vi "Color Test.vi"() -> ()   [LabVIEW 2015]
panel:
  in  "OK":bool
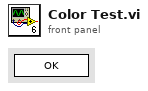
[diagram p1: front panel]
types:
  T1 = enum32{"invalid app kind", "Development System", "Run Time System", "Student Edition", "Embedded LabVIEW", "Evaluation", "Custom"}
  T2 = enum32{"Invalid", "Standard", "Closed", "Hidden", "Minimized", "Maximized"}
  T3 = cluster{"Core":cluster{"Current VI Reference":refnum<vi>, "Close Panel on Exit?":bool}, "Color data":cluster{"Attribute":string, "Color":u32}[][]}
  T4 = cluster{"Current VI Reference":refnum<vi>, "Close Panel on Exit?":bool}
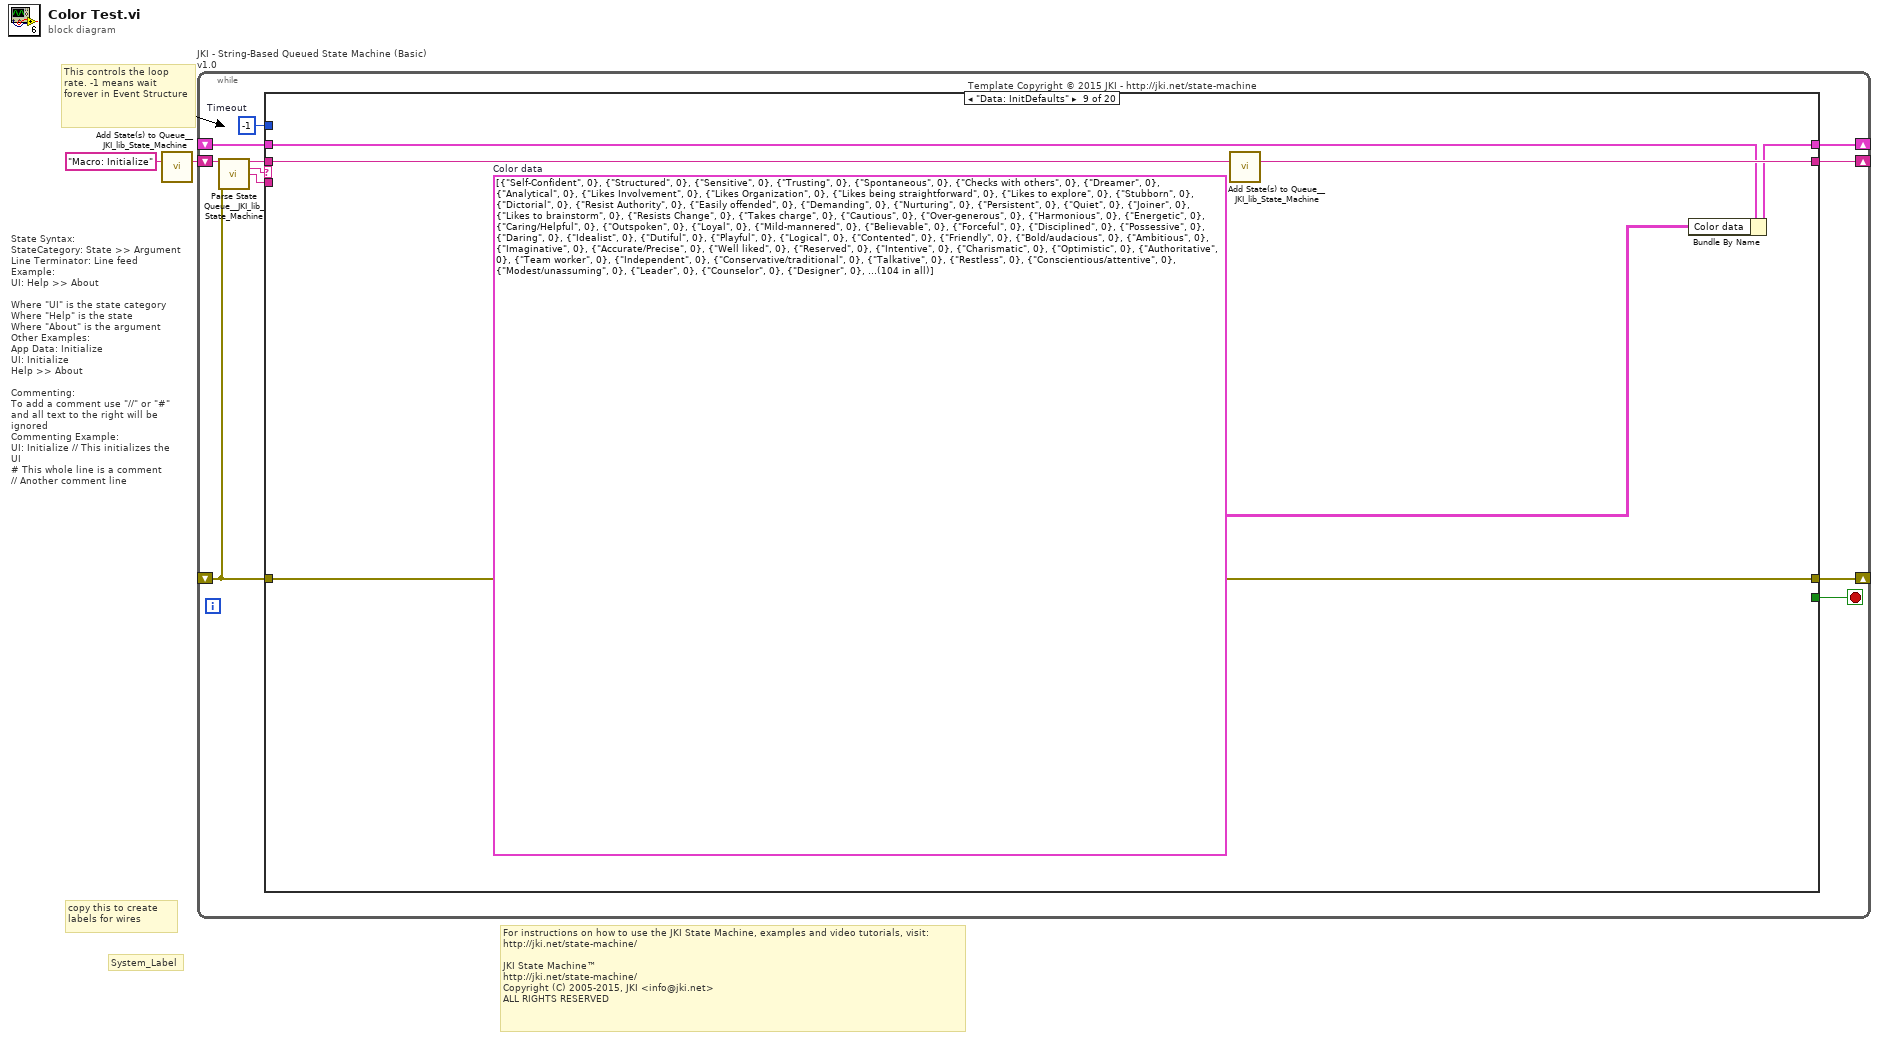
[diagram p0: block diagram]
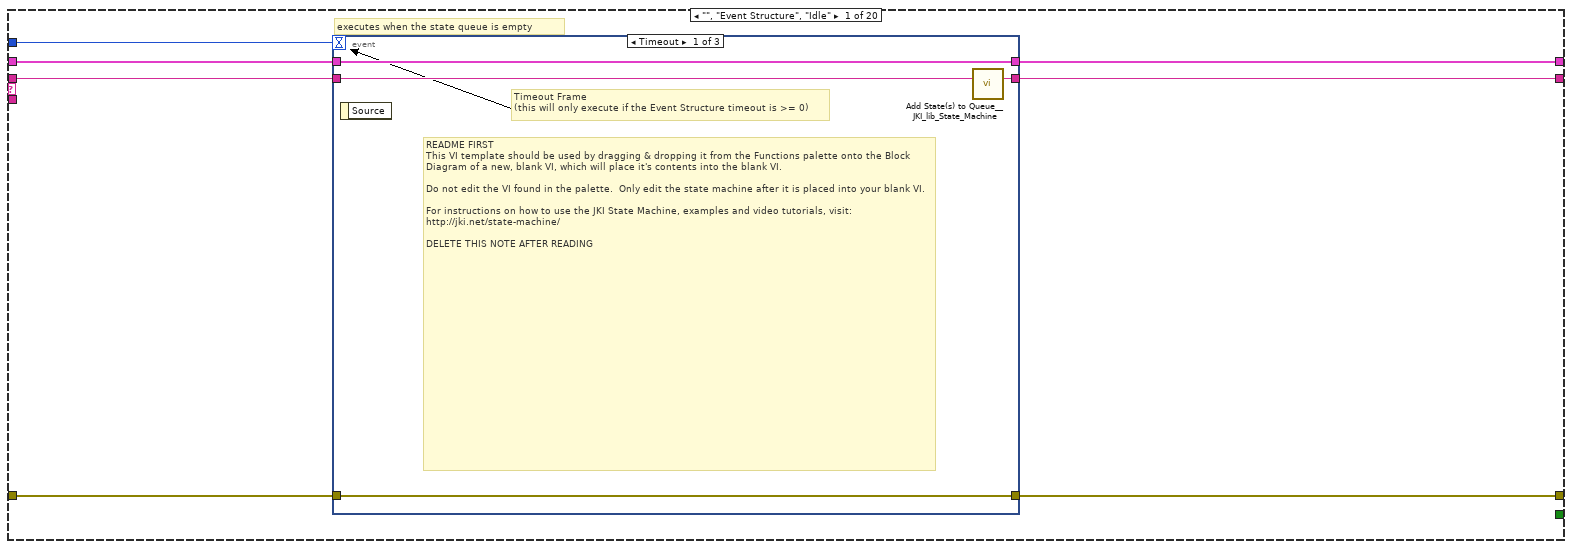
[diagram p2: hidden frame]
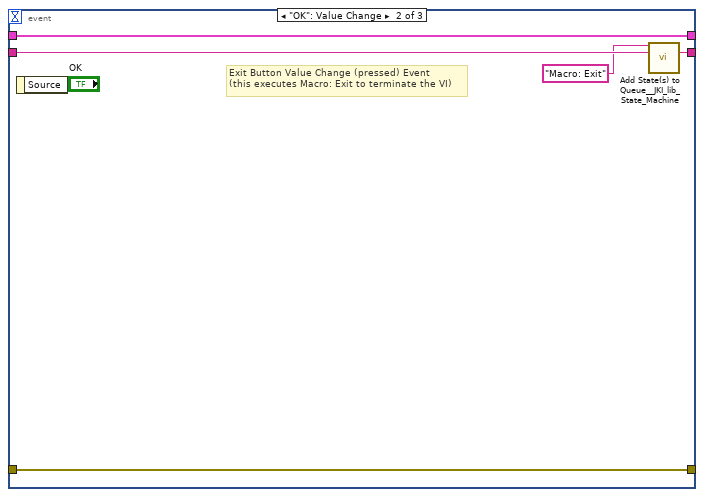
[diagram p3: hidden frame]
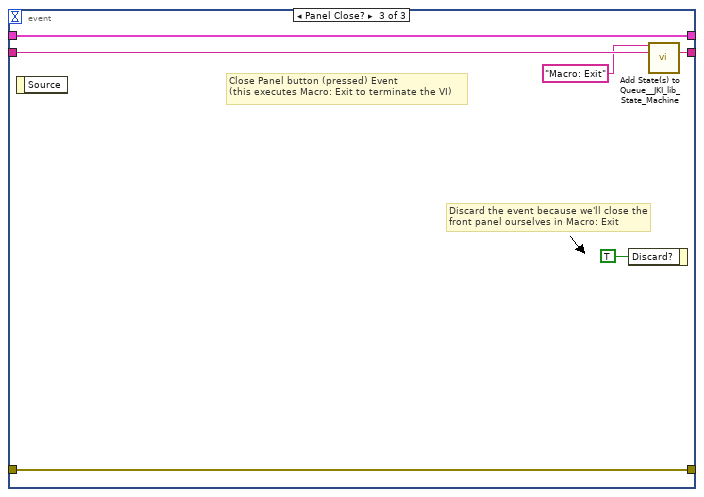
[diagram p4: hidden frame]
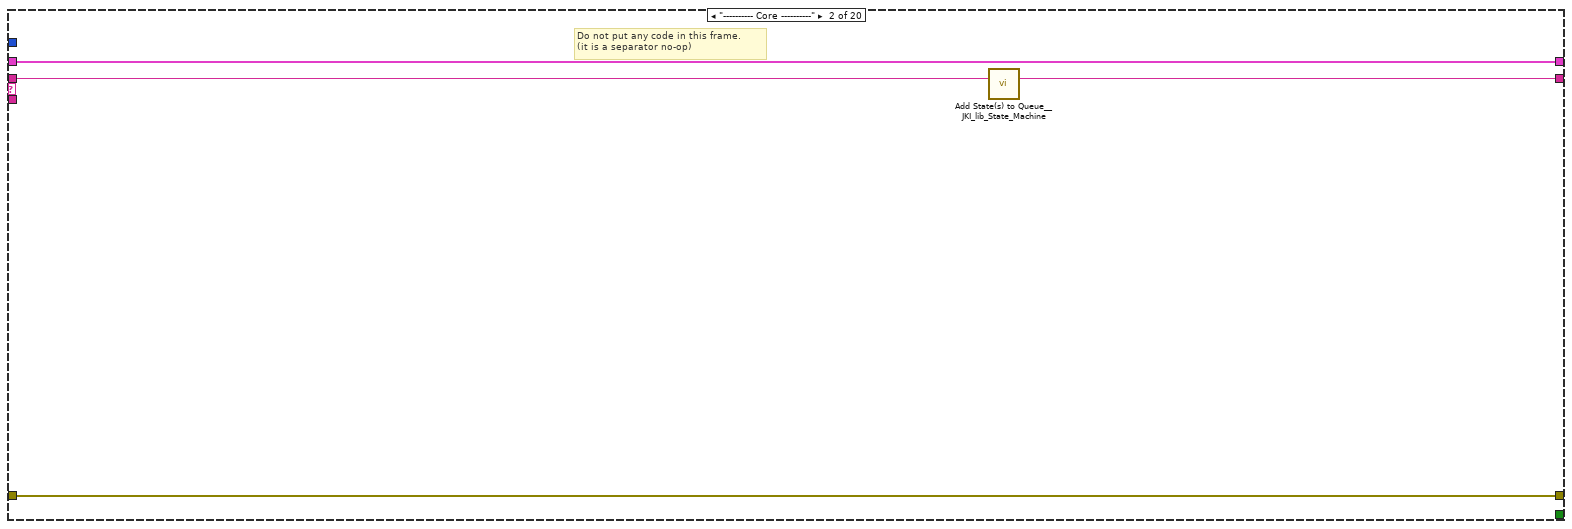
[diagram p5: hidden frame]
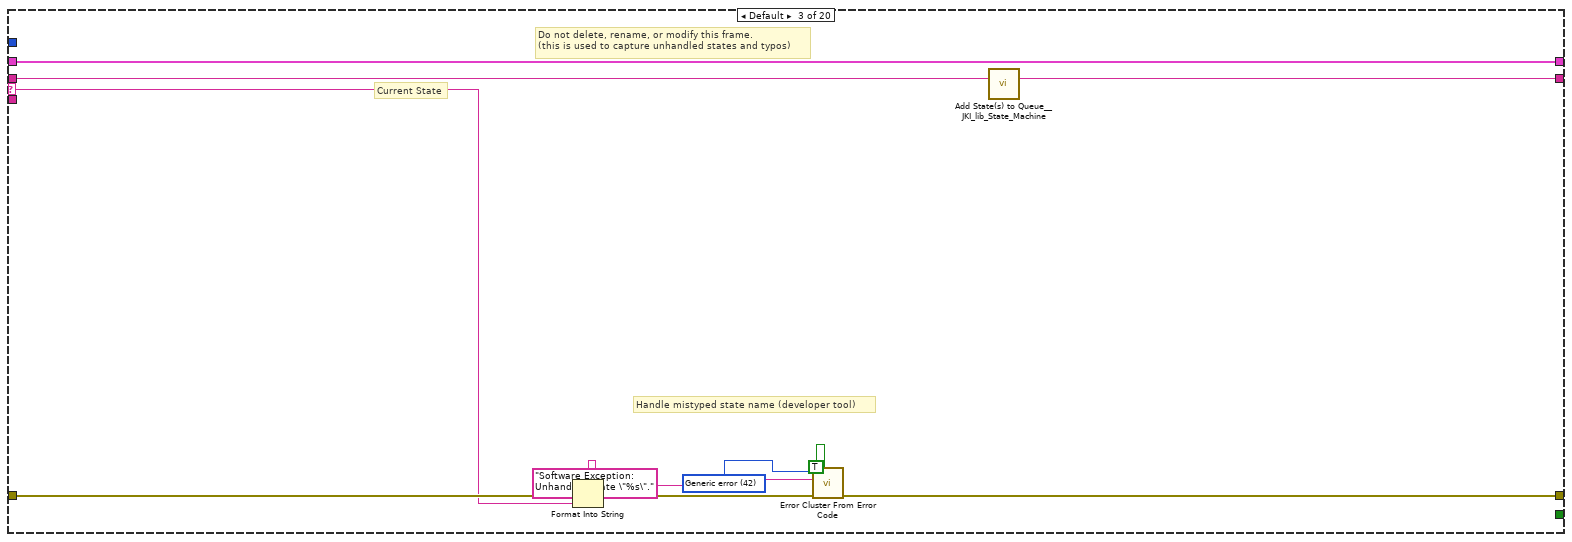
[diagram p6: hidden frame]
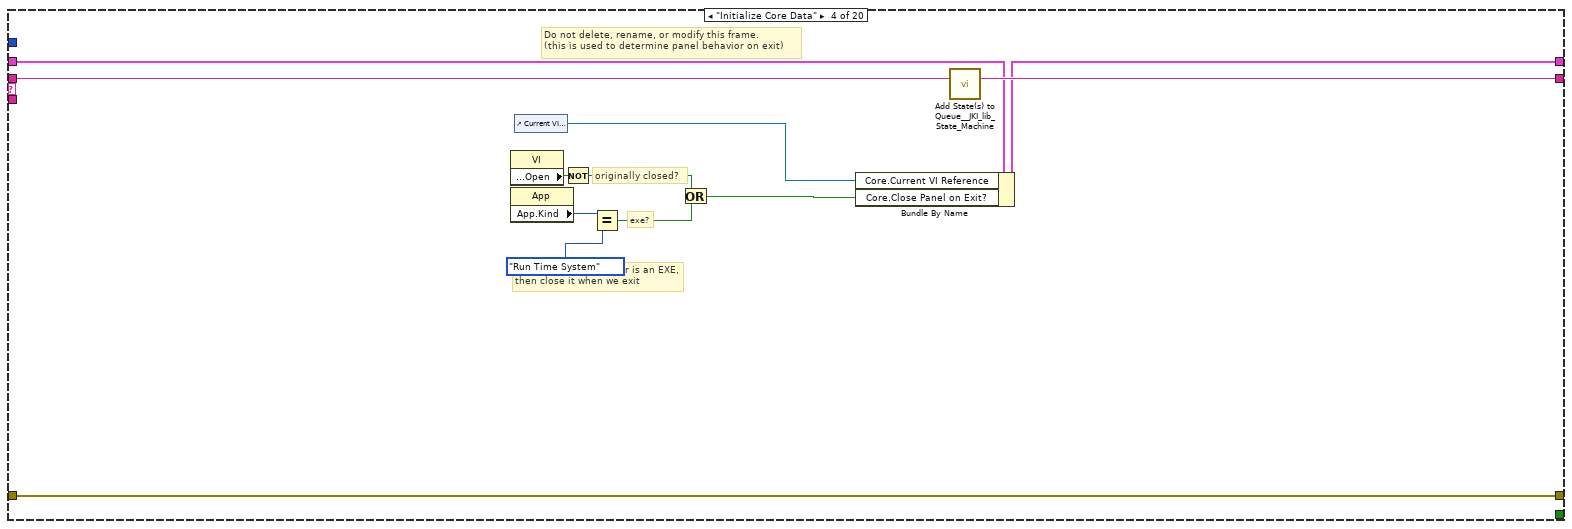
[diagram p7: hidden frame]
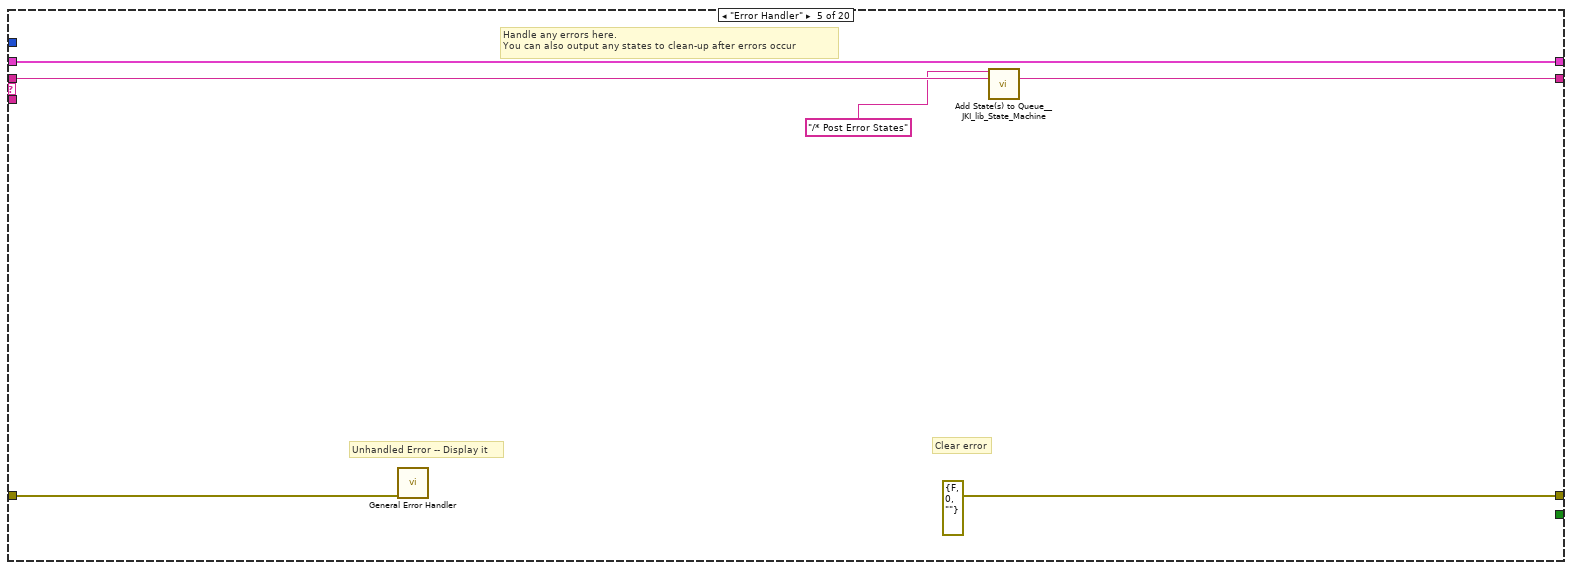
[diagram p8: hidden frame]
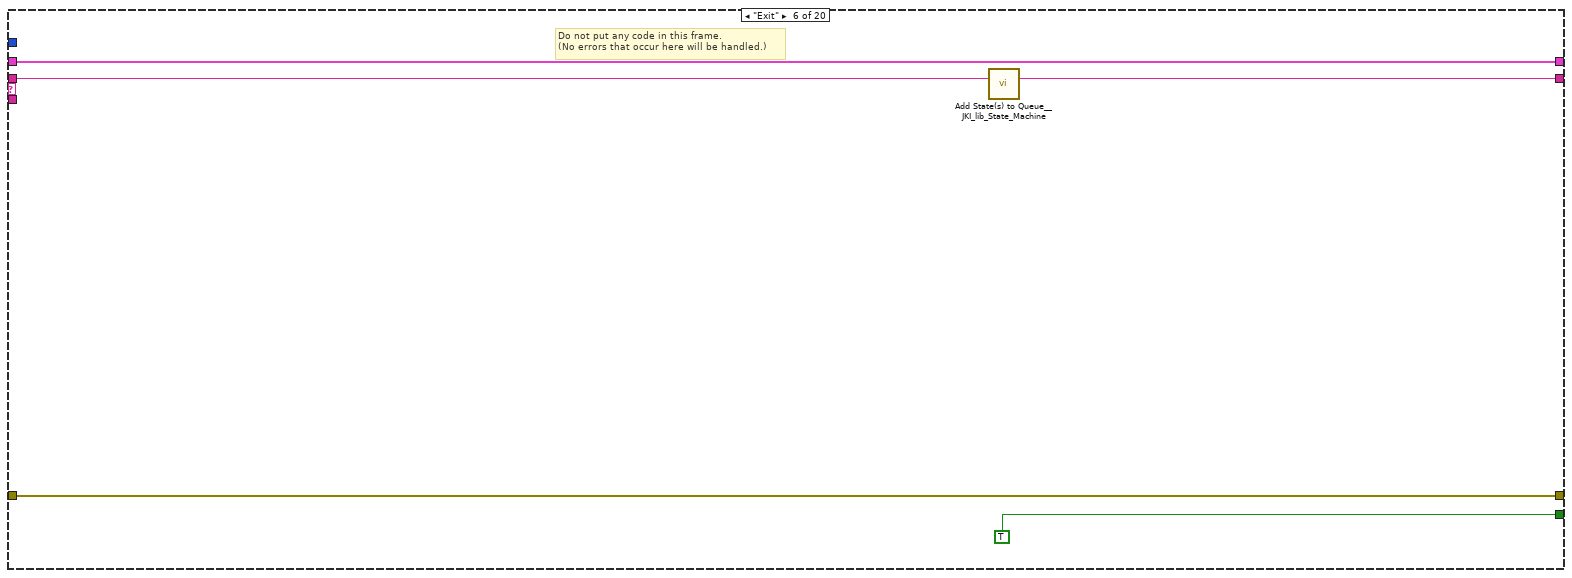
[diagram p9: hidden frame]
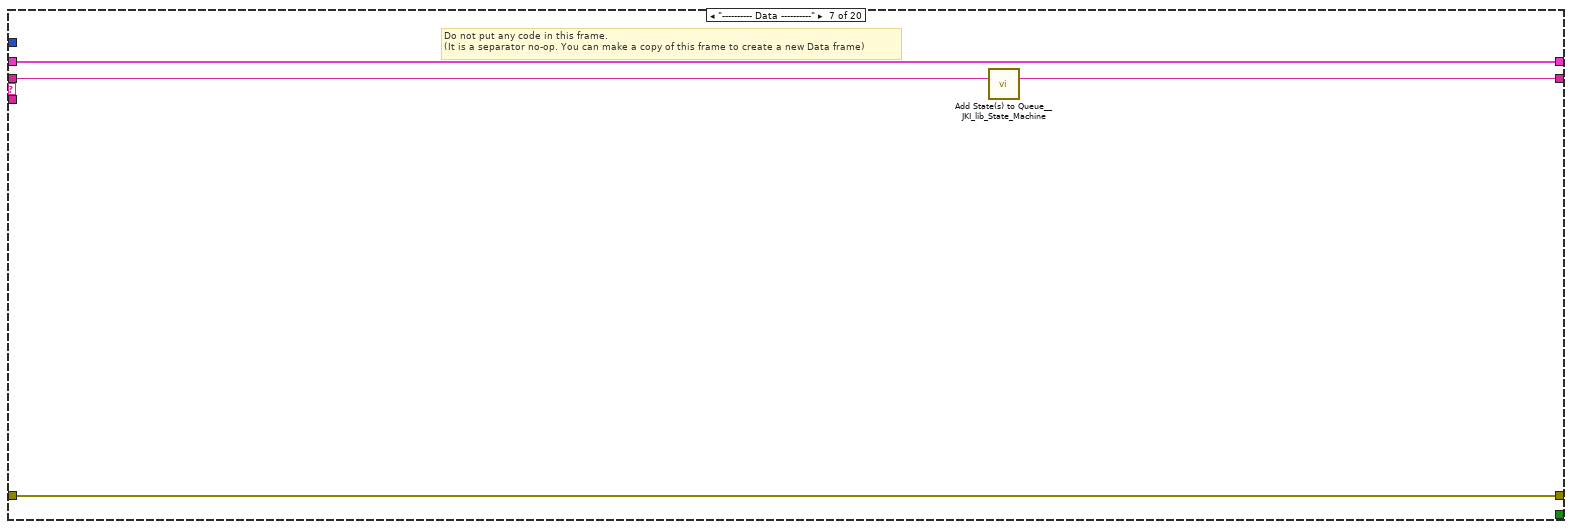
[diagram p10: hidden frame]
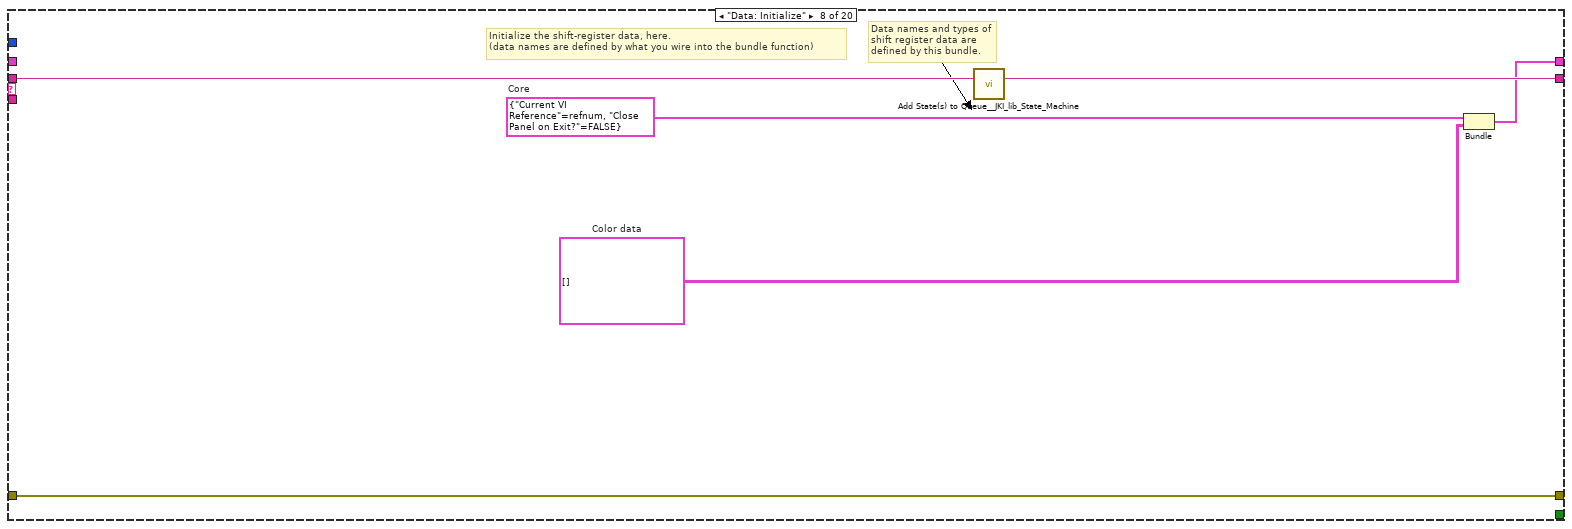
[diagram p11: hidden frame]
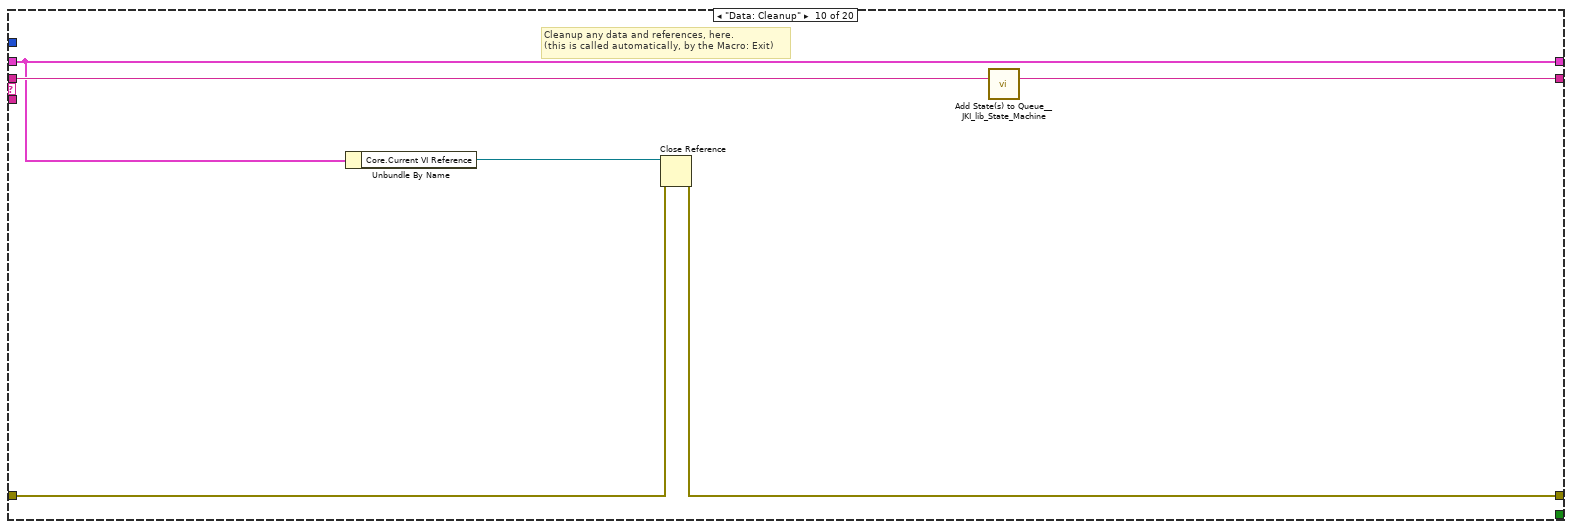
[diagram p12: hidden frame]
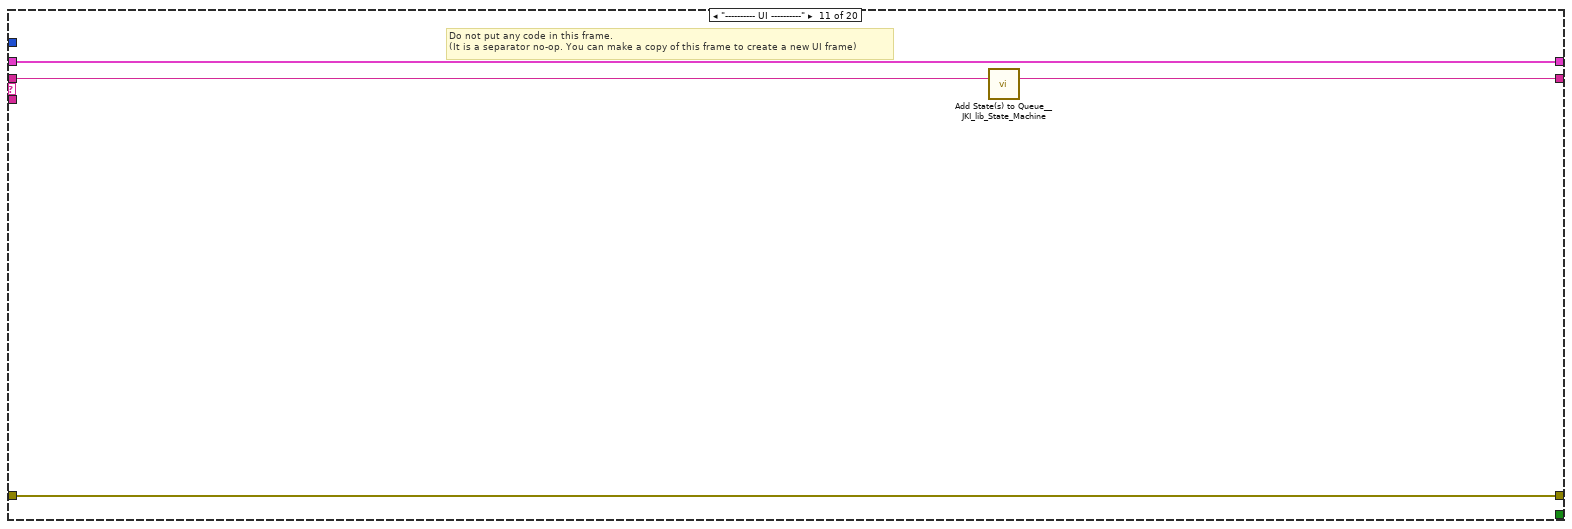
[diagram p13: hidden frame]
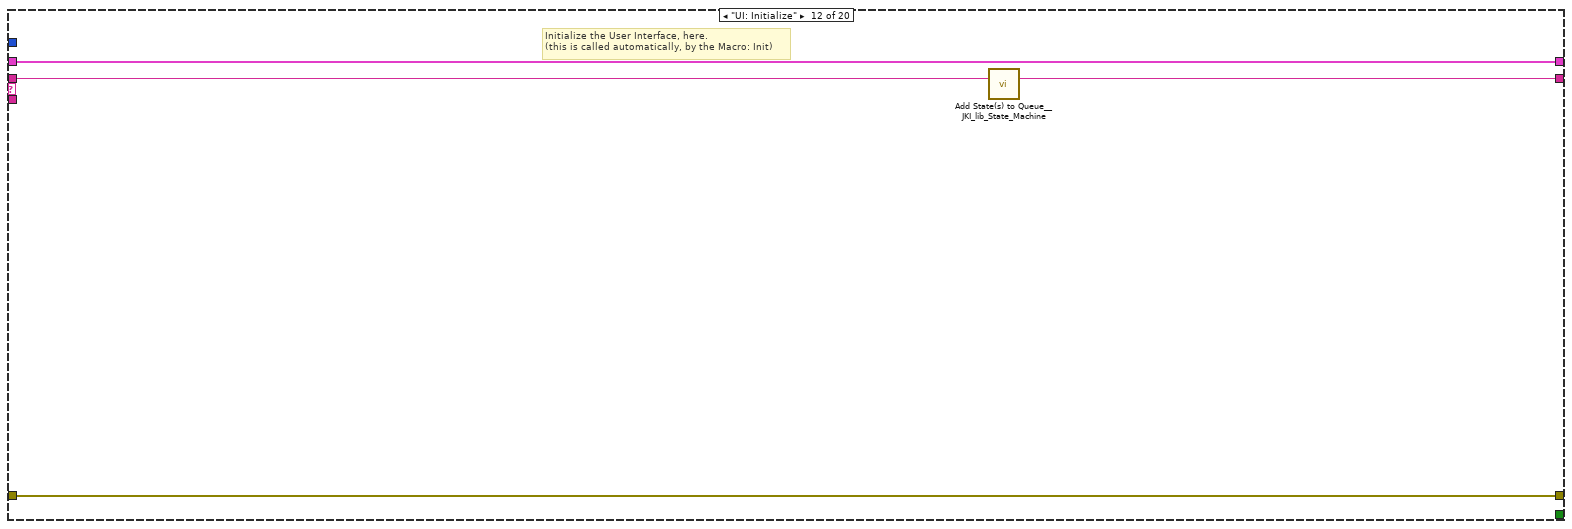
[diagram p14: hidden frame]
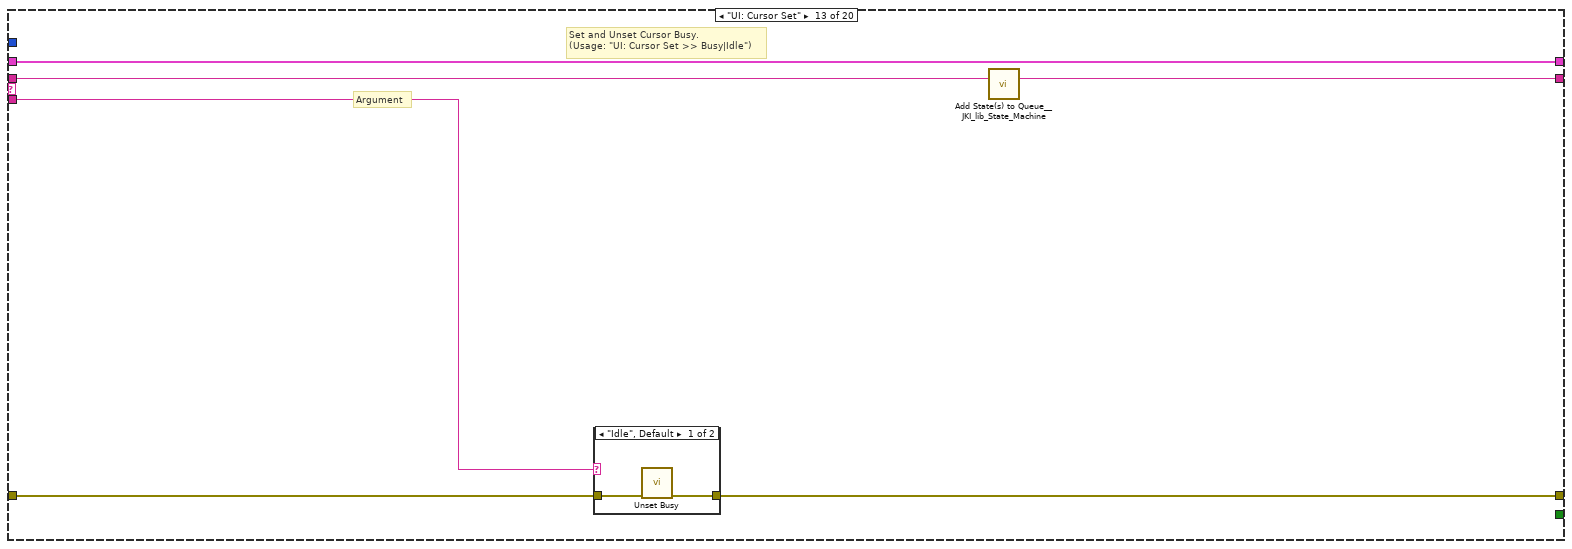
[diagram p15: hidden frame]
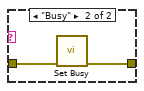
[diagram p16: hidden frame]
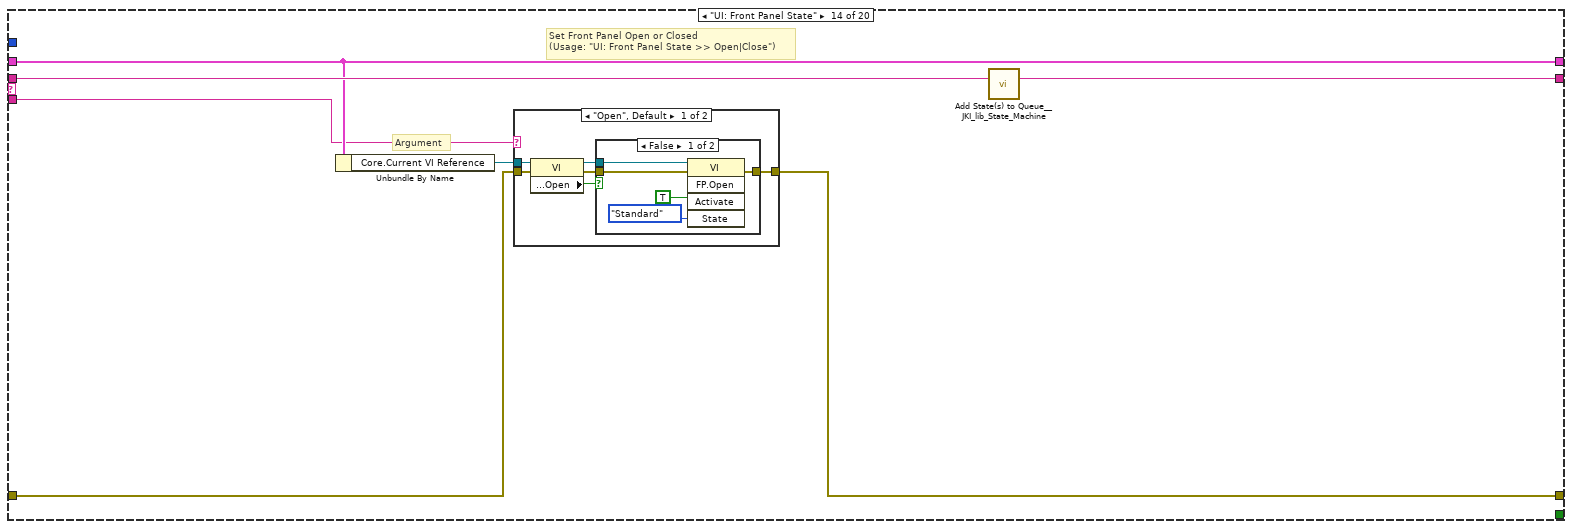
[diagram p17: hidden frame]
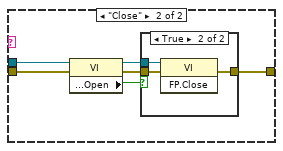
[diagram p19: hidden frame]
diagram:
  # "For instructions on how to use the JKI State Machine, examples and video tutorials, visit:\nhttp://jki.net/state-machine/\n\nJKI State Machine™\nhttp://jki.net/state-machine/\nCopyright (C) 2005-2015, JKI <info@jki.net>\nALL RIGHTS RESERVED"
  # "State Syntax:\nStateCategory: State >> Argument\nLine Terminator: Line feed\nExample:\nUI: Help >> About\n\nWhere \"UI\" is the state category\nWhere \"Help\" is the state\nWhere \"About\" is the argument\nOther Examples:\nApp Data: Initialize\nUI: Initialize\nHelp >> About\n\nCommenting:\nTo add a comment use \"//\" or \"#\" and all text to the right will be ignored\nCommenting Example:\nUI: Initialize // This initializes the UI\n# This whole line is a comment\n// Another comment line"
  # "copy this to create labels for wires"
  # "This controls the loop rate. -1 means wait forever in Event Structure"
  # "System_Label"
  n1 = call <vilib>:"Add State(s) to Queue__JKI_lib_State_Machine.vi"("State(s) in (\"\")"="Macro: Initialize") -> ("States Out"=w2:string)  [unwired: 14 in]
  n2 = while "JKI - String-Based Queued State Machine (Basic) v1.0" {
    shift-right: [w6] -> _
    shift-left: _ -> [w5]
    shift-right: [w9] -> _
    shift-left: _ -> [w3]
    shift-right: [w8] -> _
    shift-left: w2 -> [w10]
    stop <- w7 stop-if-true
    w4 = -1  # Timeout
    # "Template Copyright © 2015 JKI - http://jki.net/state-machine"
    n3 = call <vilib>:"Parse State Queue__JKI_lib_State_Machine.vi"("State Queue"=w10, "Error In (no error)"=w3) -> ("Remaining States"=w12:string, "Current State"=w13:string, "Arguments"=w11:string)  [unwired: 11 in]
    n4 = case shown="\"Data: InitDefaults\"" w13 {
      selector: w13 -> [_ _ w40 _ _ _ _ _ _ _ _ _ _ _ _ _ _ _ _ _]
      tunnel: w12 -> [w20 w39 w44 w62 w68 w73 w77 w83 w89 w95 w99 w103 w109 w120 w146 w151 w161 w165 w169 w173]
      tunnel: w11 -> [_ _ _ _ _ _ _ _ _ _ _ _ w104 w114 _ _ _ _ _ _]
      tunnel: w5 -> [w18 w36 w42 w53 w65 w71 w74 _ w86 w90 w96 w101 w107 w116 w143 w148 w158 w162 w166 w170]
      tunnel: [w17 w37 w46 w59 errorcluster {"status"=FALSE, "code"=0, "source"=""} ("error out") w70 w75 w80 w87 w91 w97 w100 w105 w117 w144 w149 w159 w163 w167 w171] -> w9
      tunnel: w3 -> [w16 w37 w45 w59 w64 w70 w75 w80 w87 w92 w97 w100 w106 w118 w144 w149 w159 w163 w167 w171]
      tunnel: [w19 w38 w43 w61 w67 w72 w76 w82 w88 w94 w98 w102 w108 w119 w145 w150 w160 w164 w168 w172] -> w8
      tunnel: [_ _ _ _ _ TRUE _ _ _ _ _ _ _ _ _ _ _ _ _ _] -> w7
      tunnel: [w15 w36 w42 w60 w65 w71 w74 w81 w85 w90 w96 w101 w107 w116 w143 w148 w158 w162 w166 w170] -> w6
      tunnel: w4 -> [w14 _ _ _ _ _ _ _ _ _ _ _ _ _ _ _ _ _ _ _]
      frame "", "Event Structure", "Idle" {
        # "executes when the state queue is empty"
        n5 = event shown="[0] Timeout" {
          selector: _ -> [_ _ _]
          dyn-events: _ -> [_ _ _]
          timeout: w14 -> [_ _ _]
          tunnel: w20 -> [w24 w29 w35]
          tunnel: [w23 w28 w34] -> w19
          tunnel: w18 -> [w21 w26 w32]
          tunnel: [w22 w27 w33] -> w17
          tunnel: w16 -> [w22 w27 w33]
          tunnel: [w21 w26 w32] -> w15
          event Timeout {
            # "README FIRST\nThis VI template should be used by dragging & dropping it from the Functions palette onto the Block Diagram of a new, blank VI, which will place it's contents into the blank VI.\n\nDo not edit the VI found in the palette.  Only edit the state machine after it is placed into your blank VI.\n\nFor instructions on how to use the JKI State Machine, examples and video tutorials, visit:\nhttp://jki.net/state-machine/\n\nDELETE THIS NOTE AFTER READING"
            # "Timeout Frame\n(this will only execute if the Event Structure timeout is >= 0)"
            n6 = event-data() -> ()  [unwired: 1 in, 1 out]
            n7 = call <vilib>:"Add State(s) to Queue__JKI_lib_State_Machine.vi"("State(s) in (\"\")"=w24) -> ("States Out"=w23:string)  [unwired: 14 in]
          }
          event "OK": Value Change {
            # "Exit Button Value Change (pressed) Event\n(this executes Macro: Exit to terminate the VI)"
            n8 = event-data() -> ()  [unwired: 1 in, 1 out]
            n9 = call <vilib>:"Add State(s) to Queue__JKI_lib_State_Machine.vi"("State(s) in Front (\"\")"="Macro: Exit", "State(s) in (\"\")"=w29) -> ("States Out"=w28:string)  [unwired: 13 in]
          }
          event Panel Close? {
            # "Discard the event because we'll close the front panel ourselves in Macro: Exit"
            # "Close Panel button (pressed) Event\n(this executes Macro: Exit to terminate the VI)"
            n10 = event-data() -> ()  [unwired: 1 in, 1 out]
            n11 = event-data("Discard?"=TRUE) -> ()  [unwired: 1 in, 1 out]
            n12 = call <vilib>:"Add State(s) to Queue__JKI_lib_State_Machine.vi"("State(s) in Front (\"\")"="Macro: Exit", "State(s) in (\"\")"=w35) -> ("States Out"=w34:string)  [unwired: 13 in]
          }
        }
      }
      frame "---------- Core ----------" {
        # "Do not put any code in this frame.\n(it is a separator no-op)"
        n13 = call <vilib>:"Add State(s) to Queue__JKI_lib_State_Machine.vi"("State(s) in (\"\")"=w39) -> ("States Out"=w38:string)  [unwired: 14 in]
      }
      frame Default {
        w49 = 42 items=["No error", "Argument error", "Memory is full", "Out of zone", "End of file", "File already open", "Generic file I/O error", "File not found", "File permission error", "Disk is full", "Duplicate path", "Too many files open", "System feature not enabled", "Resource file not found", "Cannot add resource", "Resource not found", "Image not found", "Image memory error", "Pen does not exist", "Config type invalid", "Config token not found", "Config parse error", "Config memory error", "Bad external code format", "Bad external code offset", "External code not present", "Null window", "Destroy window error", "Null menu", "Print aborted", "Bad print record", "Print driver error", "Windows error during printing", "Memory error during printing", "Print dialog error", "Generic print error", "Invalid device refnum", "Device not found", "Device parameter error", "Device unit error", "Cannot open device", "Device call aborted", "Generic error", "Cancelled by user", "Object ID too low", "Object ID too high", "Object not in heap", "Unknown heap", "Unknown object (invalid DefProc)", "Unknown object (DefProc not in table)", "Message out of range", "Invalid (null) method", "Unknown message", "Manager call not supported", "Bad address", "Network operation in progress", "Network operation timed out", "Connection is busy", "Network attribute not supported", "Network error", "Address in use", "System out of memory", "Connection aborted", "Connection refused", "Not connected", "Already connected", "Connection closed", "Initialization error (interapplication manager)", "Bad occurrence", "Wait on unbound occurrence handler", "Occurrence queue overflow", "Datalog type conflict", "Unused", "Unrecognized type (interapplication manager)", "Memory corrupt", "Failed to make temporary DLL", "Old CIN version", "Drag socket not found", "Failed to load drop-object", "Failed to register OLE object", "Failed to release OLE object", "Format specifier type mismatch", "Unknown format specifier", "Too few format specifiers", "Too many format specifiers", "Scan failed", "Newer CIN version", "Error converting to variant", "Runtime menu error", "Password tampered", "Variant attribute not found", "Incompatible variant data type", "Event data is not available", "Event Store is not present", "Occurrence is not found", "Event Queue is not created", "Event info is not available", "Refnum passed is NULL", "Error retrieving Class GUID", "Error retrieving CoClass GUID", "Error retrieving TypeLib GUID.", "Bad built application magic bytes.", "Specific driver is different from the specific driver associated with the Logical Name.", "There is no session opened to the class driver.", "Max Error", "MAX - Error with config objects", "MAX - Error loading configuration", "MAX - Group not supported"]
        # "Current State"
        # "Do not delete, rename, or modify this frame.\n(this is used to capture unhandled states and typos)"
        # "Handle mistyped state name (developer tool)"
        n14 = Format Into String(format string="Software Exception: Unhandled State \"%s\"." ("message"), error in=w45, w40) -> (resulting string=w48:string, error out=w47:errorcluster)  [unwired: 1 in]
        n15 = call <vilib>:"Error Cluster From Error Code.vi"("show call chain? (False)"=TRUE, "error in (no error)"=w47, "error message (\"\")"=w48, "error code (0)"=w49) -> ("error out"=w46:errorcluster)  [unwired: 5 in]
        n16 = call <vilib>:"Add State(s) to Queue__JKI_lib_State_Machine.vi"("State(s) in (\"\")"=w44) -> ("States Out"=w43:string)  [unwired: 14 in]
      }
      frame "Initialize Core Data" {
        # "Do not delete, rename, or modify this frame.\n(this is used to determine panel behavior on exit)"
        # "originally closed?"
        # "exe?"
        # "If panel starts closed or is an EXE, then close it when we exit"
        n17 = property class="VI"() -> ("Front Panel.Open"=w58:bool)  [unwired: 2 in, 2 out]
        n18 = property class="App"() -> ("App.Kind"=w57:T1)  [unwired: 2 in, 2 out]
        n19 = control-ref of="Current VI Reference"() -> (w51:refnum<vi>)
        n20 = Not(x=w58) -> (.not. x?=w55:bool)
        n21 = Equal?(x=w57, y=T1."Run Time System" ("Application:Kind")) -> (x = y?=w54:bool)
        n22 = Or(x=w55, y=w54) -> (x .or. y?=w52:bool)
        n23 = Bundle By Name(cluster=w53, "Core.Current VI Reference"=w51, "Core.Close Panel on Exit?"=w52) -> (w60:T3)
        n24 = call <vilib>:"Add State(s) to Queue__JKI_lib_State_Machine.vi"("State(s) in (\"\")"=w62) -> ("States Out"=w61:string)  [unwired: 14 in]
      }
      frame "Error Handler" {
        # "Unhandled Error -- Display it"
        # "Handle any errors here.\nYou can also output any states to clean-up after errors occur"
        # "Clear error"
        n25 = call <vilib>:"General Error Handler.vi"("error in (no error)"=w64) -> ()  [unwired: 10 in, 5 out]
        n26 = call <vilib>:"Add State(s) to Queue__JKI_lib_State_Machine.vi"("State(s) in Front (\"\")"="/* Post Error States", "State(s) in (\"\")"=w68) -> ("States Out"=w67:string)  [unwired: 13 in]
      }
      frame "Exit" {
        # "Do not put any code in this frame.\n(No errors that occur here will be handled.)"
        n27 = call <vilib>:"Add State(s) to Queue__JKI_lib_State_Machine.vi"("State(s) in (\"\")"=w73) -> ("States Out"=w72:string)  [unwired: 14 in]
      }
      frame "---------- Data ----------" {
        # "Do not put any code in this frame.\n(It is a separator no-op. You can make a copy of this frame to create a new Data frame)"
        n28 = call <vilib>:"Add State(s) to Queue__JKI_lib_State_Machine.vi"("State(s) in (\"\")"=w77) -> ("States Out"=w76:string)  [unwired: 14 in]
      }
      frame "Data: Initialize" {
        w78 = cluster{"Attribute":string, "Color":u32}[][] []  # Color data
        w79 = T4 {"Current VI Reference"=refnum, "Close Panel on Exit?"=FALSE}  # Core
        # "Data names and types of shift register data are defined by this bundle."
        # "Initialize the shift-register data, here.\n(data names are defined by what you wire into the bundle function)"
        n29 = call <vilib>:"Add State(s) to Queue__JKI_lib_State_Machine.vi"("State(s) in (\"\")"=w83) -> ("States Out"=w82:string)  [unwired: 14 in]
        n30 = Bundle("Core"=w79, "Color data"=w78) -> (w81:T3)  [unwired: 1 in]
      }
      frame "Data: InitDefaults" {
        w84 = cluster{"Attribute":string, "Color":u32}[][] [[{"Attribute"="Self-Confident", "Color"=0}, {"Attribute"="Structured", "Color"=0}, {"Attribute"="Sensitive", "Color"=0}, {"Attribute"="Trusting", "Color"=0}], [{"Attribute"="Spontaneous", "Color"=0}, {"Attribute"="Checks with others", "Color"=0}, {"Attribute"="Dreamer", "Color"=0}, {"Attribute"="Analytical", "Color"=0}], [{"Attribute"="Likes Involvement", "Color"=0}, {"Attribute"="Likes Organization", "Color"=0}, {"Attribute"="Likes being straightforward", "Color"=0}, {"Attribute"="Likes to explore", "Color"=0}], [{"Attribute"="Stubborn", "Color"=0}, {"Attribute"="Dictorial", "Color"=0}, {"Attribute"="Resist Authority", "Color"=0}, {"Attribute"="Easily offended", "Color"=0}], [{"Attribute"="Demanding", "Color"=0}, {"Attribute"="Nurturing", "Color"=0}, {"Attribute"="Persistent", "Color"=0}, {"Attribute"="Quiet", "Color"=0}], [{"Attribute"="Joiner", "Color"=0}, {"Attribute"="Likes to brainstorm", "Color"=0}, {"Attribute"="Resists Change", "Color"=0}, {"Attribute"="Takes charge", "Color"=0}], [{"Attribute"="Cautious", "Color"=0}, {"Attribute"="Over-generous", "Color"=0}, {"Attribute"="Harmonious", "Color"=0}, {"Attribute"="Energetic", "Color"=0}], [{"Attribute"="Caring/Helpful", "Color"=0}, {"Attribute"="Outspoken", "Color"=0}, {"Attribute"="Loyal", "Color"=0}, {"Attribute"="Mild-mannered", "Color"=0}], [{"Attribute"="Believable", "Color"=0}, {"Attribute"="Forceful", "Color"=0}, {"Attribute"="Disciplined", "Color"=0}, {"Attribute"="Possessive", "Color"=0}], [{"Attribute"="Daring", "Color"=0}, {"Attribute"="Idealist", "Color"=0}, {"Attribute"="Dutiful", "Color"=0}, {"Attribute"="Playful", "Color"=0}], [{"Attribute"="Logical", "Color"=0}, {"Attribute"="Contented", "Color"=0}, {"Attribute"="Friendly", "Color"=0}, {"Attribute"="Bold/audacious", "Color"=0}], [{"Attribute"="Ambitious", "Color"=0}, {"Attribute"="Imaginative", "Color"=0}, {"Attribute"="Accurate/Precise", "Color"=0}, {"Attribute"="Well liked", "Color"=0}], [{"Attribute"="Reserved", "Color"=0}, {"Attribute"="Intentive", "Color"=0}, {"Attribute"="Charismatic", "Color"=0}, {"Attribute"="Optimistic", "Color"=0}], [{"Attribute"="Authoritative", "Color"=0}, {"Attribute"="Team worker", "Color"=0}, {"Attribute"="Independent", "Color"=0}, {"Attribute"="Conservative/traditional", "Color"=0}], [{"Attribute"="Talkative", "Color"=0}, {"Attribute"="Restless", "Color"=0}, {"Attribute"="Conscientious/attentive", "Color"=0}, {"Attribute"="Modest/unassuming", "Color"=0}], [{"Attribute"="Leader", "Color"=0}, {"Attribute"="Counselor", "Color"=0}, {"Attribute"="Designer", "Color"=0}, {"Attribute"="Controller", "Color"=0}], [{"Attribute"="Meticulous", "Color"=0}, {"Attribute"="Workaholic", "Color"=0}, {"Attribute"="Supportive", "Color"=0}, {"Attribute"="Self-directed", "Color"=0}], [{"Attribute"="Industrious", "Color"=0}, {"Attribute"="Attentive to details", "Color"=0}, {"Attribute"="Prolific mental imager", "Color"=0}, {"Attribute"="Positive thinker", "Color"=0}], [{"Attribute"="Task-oriented", "Color"=0}, {"Attribute"="People-oriented", "Color"=0}, {"Attribute"="Idea-oriented", "Color"=0}, {"Attribute"="Result-oriented", "Color"=0}], [{"Attribute"="Emotional", "Color"=0}, {"Attribute"="Flexible/adaptable", "Color"=0}, {"Attribute"="Likes recognition", "Color"=0}, {"Attribute"="Particular", "Color"=0}], [{"Attribute"="Irritable", "Color"=0}, {"Attribute"="Rigid", "Color"=0}, {"Attribute"="Easily slighted", "Color"=0}, {"Attribute"="Easilythreatened", "Color"=0}], [{"Attribute"="Indirect", "Color"=0}, {"Attribute"="Frank/candid", "Color"=0}, {"Attribute"="Careful", "Color"=0}, {"Attribute"="Strict", "Color"=0}], [{"Attribute"="Goal-oriented", "Color"=0}, {"Attribute"="Capable", "Color"=0}, {"Attribute"="Volunteers for tasks", "Color"=0}, {"Attribute"="Schedule-oriented", "Color"=0}], [{"Attribute"="Excels in emergencies", "Color"=0}, {"Attribute"="Thrives on compliments", "Color"=0}, {"Attribute"="Dry sense of humour", "Color"=0}, {"Attribute"="Avoids causing attention", "Color"=0}], [{"Attribute"="Enjoys watching people", "Color"=0}, {"Attribute"="Strong-willed", "Color"=0}, {"Attribute"="Determined enthusiastic", "Color"=0}, {"Attribute"="Sets very high standards", "Color"=0}], [{"Attribute"="Very self-confident", "Color"=0}, {"Attribute"="", "Color"=0}, {"Attribute"="", "Color"=0}, {"Attribute"="", "Color"=0}]]  # Color data
        n31 = call <vilib>:"Add State(s) to Queue__JKI_lib_State_Machine.vi"("State(s) in (\"\")"=w89) -> ("States Out"=w88:string)  [unwired: 14 in]
        n32 = Bundle By Name(cluster=w86, "Color data"=w84) -> (w85:T3)
      }
      frame "Data: Cleanup" {
        # "Cleanup any data and references, here.\n(this is called automatically, by the Macro: Exit)"
        n33 = Unbundle By Name(w90) -> ("Core.Current VI Reference"=w93:refnum<vi>)
        n34 = Close Reference(reference=w93, error in (no error)=w92) -> (error out=w91:errorcluster)
        n35 = call <vilib>:"Add State(s) to Queue__JKI_lib_State_Machine.vi"("State(s) in (\"\")"=w95) -> ("States Out"=w94:string)  [unwired: 14 in]
      }
      frame "---------- UI ----------" {
        # "Do not put any code in this frame.\n(It is a separator no-op. You can make a copy of this frame to create a new UI frame)"
        n36 = call <vilib>:"Add State(s) to Queue__JKI_lib_State_Machine.vi"("State(s) in (\"\")"=w99) -> ("States Out"=w98:string)  [unwired: 14 in]
      }
      frame "UI: Initialize" {
        # "Initialize the User Interface, here.\n(this is called automatically, by the Macro: Init)"
        n37 = call <vilib>:"Add State(s) to Queue__JKI_lib_State_Machine.vi"("State(s) in (\"\")"=w103) -> ("States Out"=w102:string)  [unwired: 14 in]
      }
      frame "UI: Cursor Set" {
        # "Argument"
        # "Set and Unset Cursor Busy.\n(Usage: \"UI: Cursor Set >> Busy|Idle\")"
        n38 = case shown="\"Idle\", Default" w104 {
          tunnel: w106 -> [w111 w113]
          tunnel: [w110 w112] -> w105
          frame "Idle", Default {
            n39 = call <vilib>:"Unset Busy.vi"("error in (no error)"=w111) -> ("error out"=w110:errorcluster)  [unwired: 10 in]
          }
          frame "Busy" {
            n40 = call <vilib>:"Set Busy.vi"("error in (no error)"=w113) -> ("error out"=w112:errorcluster)  [unwired: 9 in, 1 out]
          }
        }
        n41 = call <vilib>:"Add State(s) to Queue__JKI_lib_State_Machine.vi"("State(s) in (\"\")"=w109) -> ("States Out"=w108:string)  [unwired: 14 in]
      }
      frame "UI: Front Panel State" {
        # "Argument"
        # "Set Front Panel Open or Closed\n(Usage: \"UI: Front Panel State >> Open|Close\")"
        n42 = Unbundle By Name(w116) -> ("Core.Current VI Reference"=w115:refnum<vi>)
        n43 = case shown="\"Open\", Default" w114 {
          tunnel: w118 -> [w124 w137]
          tunnel: [w126 w138] -> w117
          tunnel: w115 -> [w125 w135]
          frame "Open", Default {
            n44 = property class="VI"(reference=w125, error in=w124) -> (reference out=w122:refnum<vi>, error out=w123:errorcluster, "Front Panel.Open"=w121:bool)
            n45 = case shown="False" w121 {
              tunnel: [w129 w132] -> w126
              tunnel: w123 -> [w128 w132]
              tunnel: w122 -> [w127 _]
              frame False {
                n46 = invoke class="VI" method="FP.Open"(reference=w127, error in=w128, "Activate"=TRUE, "State"=T2."Standard") -> (error out=w129:errorcluster)  [unwired: 1 in, 4 out]
              }
              frame True {
              }
            }
          }
          frame "Close" {
            n47 = property class="VI"(reference=w135, error in=w137) -> (reference out=w134:refnum<vi>, error out=w136:errorcluster, "Front Panel.Open"=w133:bool)
            n48 = case shown="True" w133 {
              tunnel: [w139 w142] -> w138
              tunnel: w136 -> [w139 w141]
              tunnel: w134 -> [_ w140]
              frame False {
              }
              frame True {
                n49 = invoke class="VI" method="FP.Close"(reference=w140, error in=w141) -> (error out=w142:errorcluster)  [unwired: 1 in, 2 out]
              }
            }
          }
        }
        n50 = call <vilib>:"Add State(s) to Queue__JKI_lib_State_Machine.vi"("State(s) in (\"\")"=w120) -> ("States Out"=w119:string)  [unwired: 14 in]
      }
      frame "---------- Macro ----------" {
        # "Do not put any code in this frame.\n(It is a separator no-op. You can make a copy of this frame to create a new Macro frame)"
        n51 = call <vilib>:"Add State(s) to Queue__JKI_lib_State_Machine.vi"("State(s) in (\"\")"=w146) -> ("States Out"=w145:string)  [unwired: 14 in]
      }
      frame "Macro: Initialize" {
        w147 = "Data: Initialize\nData: InitDefaults\nInitialize Core Data\nUI: Initialize\nUI: Front Panel State >> Open"  # Data: Initialize Data: InitDefaults Initialize Core Data UI: Initialize UI: Front Panel State >> Open
        # "Initialization Macro\n(This is called once, when the VI starts)"
        n52 = call <vilib>:"Add State(s) to Queue__JKI_lib_State_Machine.vi"("State(s) in Front (\"\")"=w147, "State(s) in (\"\")"=w151) -> ("States Out"=w150:string)  [unwired: 13 in]
      }
      frame "Macro: Exit" {
        # "Exit Macro\n(This is called once, when the VI exits)"
        n53 = Unbundle By Name(w158) -> ("Core.Close Panel on Exit?"=w157:bool)
        n54 = Select(t="UI: Front Panel State >> Close", s=w157, f="") -> (s? t:f=w154:string)
        n55 = call <vilib>:"Add State(s) to Queue__JKI_lib_State_Machine.vi"("State(s) in (\"\")"=w154, "State(s) at Back (\"\")"="Data: Cleanup\nExit") -> ("States Out"=w152:string)  [unwired: 13 in]
        n56 = call <vilib>:"Add State(s) to Queue__JKI_lib_State_Machine.vi"("State(s) in Front (\"\")"=w152, "State(s) in (\"\")"=w161) -> ("States Out"=w160:string)  [unwired: 13 in]
      }
      frame "---------- New Category ----------" {
        # "Template Separator\n(You can make a copy of, or modify, this frame)"
        n57 = call <vilib>:"Add State(s) to Queue__JKI_lib_State_Machine.vi"("State(s) in (\"\")"=w165) -> ("States Out"=w164:string)  [unwired: 14 in]
      }
      frame "New Category: 1" {
        # "Your code here.\n(You can make a copy of, or modify, this frame)"
        n58 = call <vilib>:"Add State(s) to Queue__JKI_lib_State_Machine.vi"("State(s) in (\"\")"=w169) -> ("States Out"=w168:string)  [unwired: 14 in]
      }
      frame "New Category: 2" {
        # "Your code here.\n(You can make a copy of, or modify, this frame)"
        n59 = call <vilib>:"Add State(s) to Queue__JKI_lib_State_Machine.vi"("State(s) in (\"\")"=w173) -> ("States Out"=w172:string)  [unwired: 14 in]
      }
    }
  }
